vi "Upload.vi"(7 "Node-ID":u8, 10 "Multiplexer":cluster{"Index":u16, "Sub-Index":u8} {"Sub-Index" format="%.0x"; "Index" format="%.0x"}, 11 "Service Data Object in":refnum<class "Service Data Object.lvclass">) -> (1 "Request":refnum<class "CANopen Request Message.lvclass">, 2 "Expected Response":refnum<class "CANopen Response Message.lvclass">, 3 "Service Data Object out":refnum<class "Service Data Object.lvclass">)   [LabVIEW 2024, in "CANopen Master.lvlib" / "Service Data Object.lvclass"]
uses:
  Service Data Object.lvclass
  CANopen Request/CANopen Request Message.lvclass
  CANopen Response/CANopen Response Message.lvclass
  CANopen/FunctionCode.ctl
  Initiate Down-Upload Response Comparator/Initiate Down-Upload Response Comparator.lvclass
  Service Data Object.lvclass/Service Data Object.ctl
  SDO Response Compare Strategy/SDO Response Compare Strategy.lvclass/SDO Response Compare Strategy.ctl
  CANopen Master.lvlib
  CANopen Message/CANopen Message.lvclass
  SDO Response Compare Strategy/SDO Response Compare Strategy.lvclass
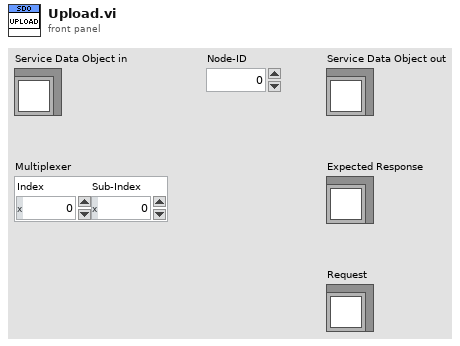
[diagram p1: front panel]
types:
  T1 = typedef "CANopen Master.lvlib/FunctionCode.ctl" = u16
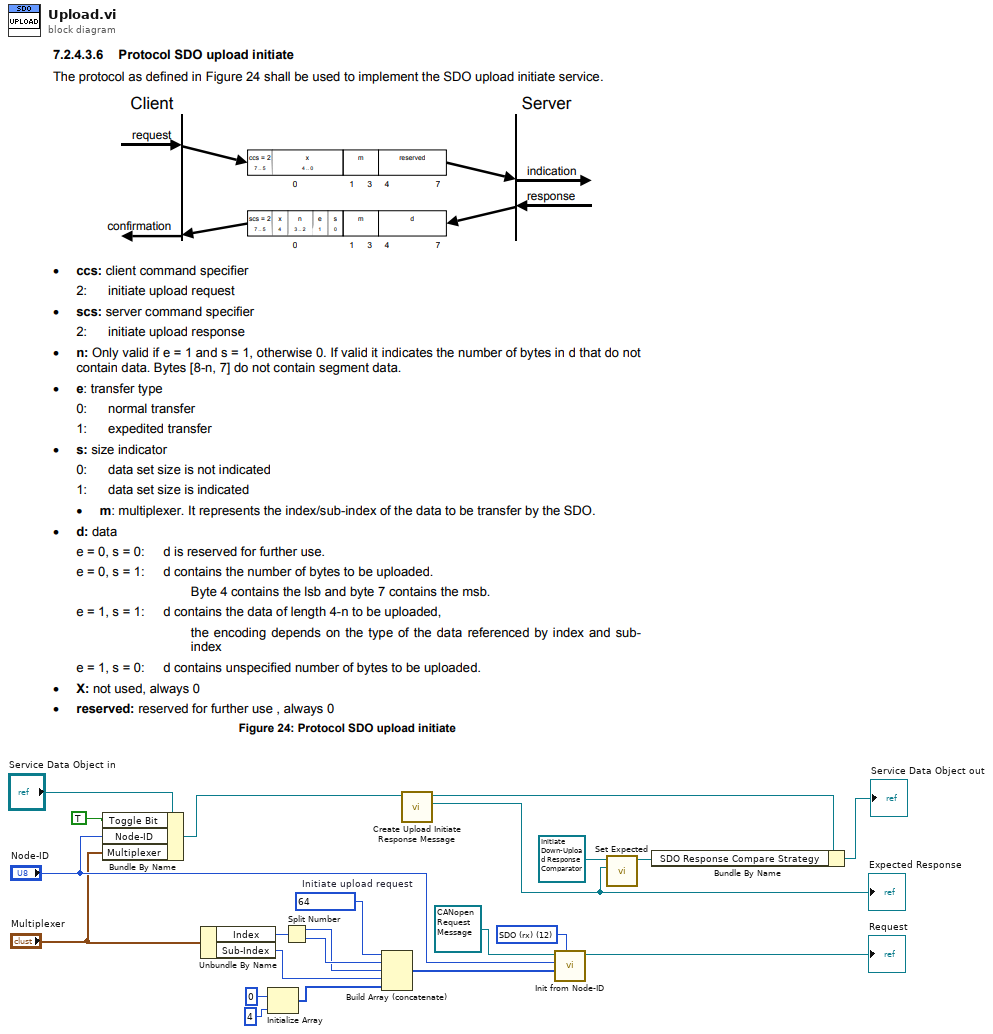
[diagram p0: block diagram]
diagram:
  w15 = T1 12 items=["EMCY"=1, "PDO1 (tx)"=3, "PDO1 (rx)"=4, "PDO2 (tx)"=5, "PDO2 (rx)"=6, "PDO3 (tx)"=7, "PDO3 (rx)"=8, "PDO4 (tx)"=9, "PDO4 (rx)"=10, "SDO (tx)"=11, "SDO (rx)"=12, "NMT error control"=14] ("Function code")
  w13 = u8 64  # Initiate upload request
  n1 = Bundle By Name(cluster="Service Data Object in", "Toggle Bit"=TRUE, "Node-ID"="Node-ID", "Multiplexer"="Multiplexer") -> (w9:refnum<class "Service Data Object.lvclass">)
  n2 = Unbundle By Name("Multiplexer") -> ("Index"=w22:u16, "Sub-Index"=w19:u8)
  n3 = Initialize Array(u8 0, 4 ("y")) -> (w17:u8[])
  n4 = Split Number(x=w22) -> (hi(x)=w20:u8, lo(x)=w21:u8)
  n5 = Build Array (concatenate)(w13, w21, w20, w19, w17) -> (w14:u8[])
  n6 = call "Create Upload Initiate Response Message.vi"("Service Data Object in"=w9) -> ("Response Message"=w3:refnum<class "CANopen Response Message.lvclass">, "Service Data Object out"=w5:refnum<class "Service Data Object.lvclass">)  [unwired: 9 in]
  "Expected Response" <- w3
  n7 = call "Init from Node-ID.vi"("Function code"=w15, "Data"=w14, "Node-ID"="Node-ID", "CANopen Message in"=refnum<class "CANopen Request Message.lvclass"> refnum ("CANopen Master.lvlib:CANopen Request Message.lvclass")) -> ("CANopen Message out"=→"Request":refnum<class "CANopen Request Message.lvclass">)  [unwired: 7 in]
  n8 = call "Set Expected.vi"("CANopen Message"=w3, "SDO Response Compare Strategy in"=refnum<class "Initiate Down-Upload Response Comparator.lvclass"> refnum ("CANopen Master.lvlib:Initiate Down-Upload Response Comparator.lvclass")) -> ("SDO Response Compare Strategy out"=w6:refnum<class "Initiate Down-Upload Response Comparator.lvclass">)  [unwired: 9 in]
  n9 = Bundle By Name(cluster=w5, "SDO Response Compare Strategy"=w6) -> (→"Service Data Object out":refnum<class "Service Data Object.lvclass">)
